vi "Registered Messages.vi"() -> (3 "registered messages":string[](array[string]))   [LabVIEW 2021, in "TemplateProcess.lvlib"]
uses:
  TemplateProcess.lvlib
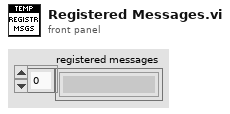
[diagram p1: front panel]
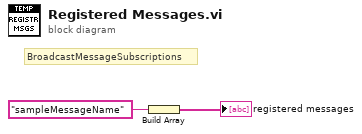
[diagram p0: block diagram]
diagram:
  # "BroadcastMessageSubscriptions"
  n1 = Build Array("sampleMessageName" ("String")) -> (→"registered messages":string[])
